vi "Read Output.vi"(0 "VISA resource name":refnum<visa-resource-name>, 11 "error in (no error)":errorcluster) -> (4 "VISA resource name out":refnum<visa-resource-name>, 6 "Actual Voltage Level (V)":dbl format="%.4g", 8 "Actual Current Level (A)":dbl format="%.4g", 10 "Actual Power Level (W)":dbl format="%.4g", 15 "error out":errorcluster)   [LabVIEW 2021, in "BK Precision 9200 Series.lvlib"]
doc: "Returns the actual voltage, current, and power level of the output."
uses:
  <instrlib>/BK Precision 9200 Series/BK Precision 9200 Series.lvlib
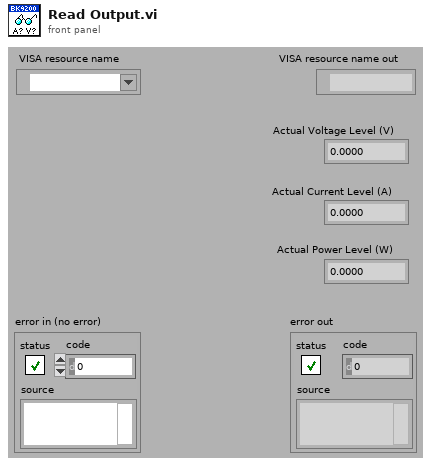
[diagram p1: front panel]
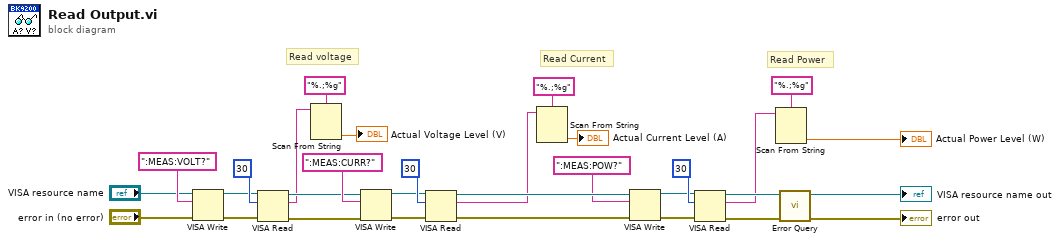
[diagram p0: block diagram]
diagram:
  # "Read Power"
  # "Read Current"
  # "Read voltage"
  n1 = VISA Write(VISA resource name="VISA resource name", write buffer=":MEAS:VOLT?", error in (no error)="error in (no error)") -> (VISA resource name out=w27:refnum<visa-resource-name>, error out=w26:errorcluster)  [unwired: 1 out]
  n2 = VISA Read(VISA resource name=w27, byte count=30, error in (no error)=w26) -> (VISA resource name out=w21:refnum<visa-resource-name>, read buffer=w6:string, error out=w20:errorcluster)  [unwired: 1 out]
  n3 = Scan From String(format string="%.;%g", input string=w6) -> (output 1=→"Actual Voltage Level (V)":dbl)  [unwired: 3 in, 3 out]
  n4 = VISA Write(VISA resource name=w21, write buffer=":MEAS:CURR?", error in (no error)=w20) -> (VISA resource name out=w23:refnum<visa-resource-name>, error out=w22:errorcluster)  [unwired: 1 out]
  n5 = VISA Read(VISA resource name=w23, byte count=30, error in (no error)=w22) -> (VISA resource name out=w14:refnum<visa-resource-name>, read buffer=w5:string, error out=w13:errorcluster)  [unwired: 1 out]
  n6 = Scan From String(format string="%.;%g", input string=w5) -> (output 1=→"Actual Current Level (A)":dbl)  [unwired: 3 in, 3 out]
  n7 = VISA Write(VISA resource name=w14, write buffer=":MEAS:POW?", error in (no error)=w13) -> (VISA resource name out=w16:refnum<visa-resource-name>, error out=w15:errorcluster)  [unwired: 1 out]
  n8 = VISA Read(VISA resource name=w16, byte count=30, error in (no error)=w15) -> (VISA resource name out=w10:refnum<visa-resource-name>, read buffer=w4:string, error out=w11:errorcluster)  [unwired: 1 out]
  n9 = Scan From String(format string="%.;%g", input string=w4) -> (output 1=→"Actual Power Level (W)":dbl)  [unwired: 3 in, 3 out]
  n10 = call <instrlib>:"Error Query.vi"("error in (no error)"=w11, "VISA resource name"=w10) -> ("error out"=→"error out":errorcluster, "VISA resource name out"=→"VISA resource name out":refnum<visa-resource-name>)  [unwired: 6 in, 2 out]
